vi "Config Dev Span.vi"(8 "error in":errorcluster, 9 "Loss (0.2 jpF)":dbl=0.2 min=-1900.0 max=19000.0 format="%#_10f", 10 "Capacitance (2.0 pF)":dbl=2.0 min=-165000.0 max=1650000.0 format="%#_10f", 11 "VISA resource name":refnum<visa-resource-name>) -> (0 "error out":errorcluster, 3 "VISA resource name out":refnum<visa-resource-name>)   [LabVIEW 2014, in "Andeen-Hagerling 2700.lvlib"]
doc: "This VI sets the distance between the upper and lower bounds of the input deviation capacitance and loss spans in pF and jpF respectively. These deviation spans correspond directly to the analog output voltage spans for capacitance and loss respectively.\n\nThe maximum permitted value for each DSpan parameters is 600 pF, or 6% of the corresponding DPoint\nparameter value, whichever is larger. These limits are checked during the initialization of the deviation subsystem, usually upon execution of the DEV MODE ON command. If either of the DSpan setting exceeds its limit, then a DEV SPAN TOO BIG error message will be reported."
uses:
  Andeen-Hagerling 2700.lvlib
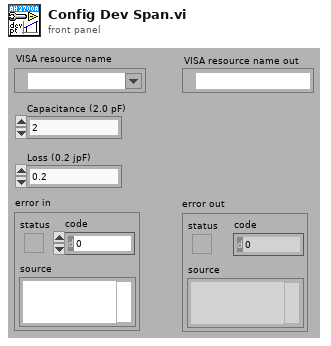
[diagram p1: front panel]
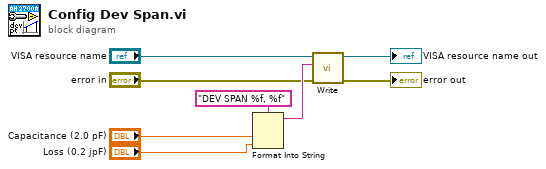
[diagram p0: block diagram]
diagram:
  n1 = Format Into String(format string="DEV SPAN %f, %f", "Capacitance (2.0 pF)", "Loss (0.2 jpF)") -> (resulting string=w7:string)  [unwired: 2 in, 1 out]
  n2 = call "Write.vi"("error in"="error in", "command"=w7, "VISA resource name"="VISA resource name") -> ("error out"=→"error out":errorcluster, "VISA resource name out"=→"VISA resource name out":refnum<visa-resource-name>)  [unwired: 7 in]
